vi "write_params.vi"(8 "error in (no error)":errorcluster, 10 "params":T1={"n_components"=2.0, "algorithm"="randomized", "n_iter"=5.0, "random_state"=0.0, "tol"=0.0}, 11 "TruncatedSVD in":refnum<class "TruncatedSVD.lvclass">) -> (0 "error out":errorcluster, 3 "TruncatedSVD out":refnum<class "TruncatedSVD.lvclass">)   [LabVIEW 2020, in "TruncatedSVD.lvclass"]
uses:
  TruncatedSVD.lvclass
  Controls/truncated_svd_params.ctl
  TruncatedSVD.lvclass/TruncatedSVD.ctl
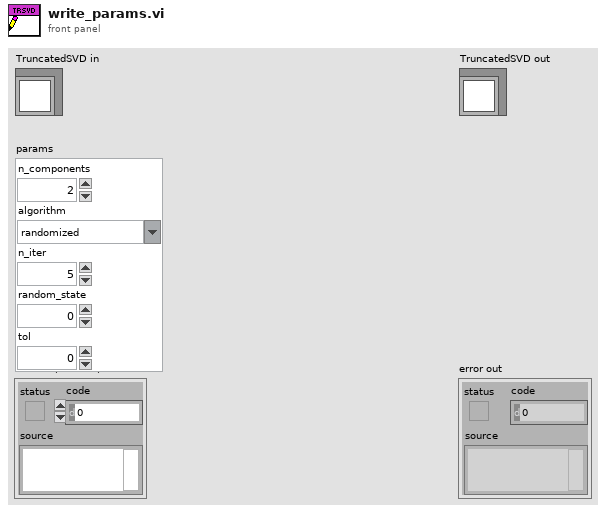
[diagram p1: front panel]
types:
  T1 = typedef "truncated_svd_params.ctl" = cluster{"n_components":dbl, "algorithm":string, "n_iter":dbl, "random_state":dbl, "tol":dbl}
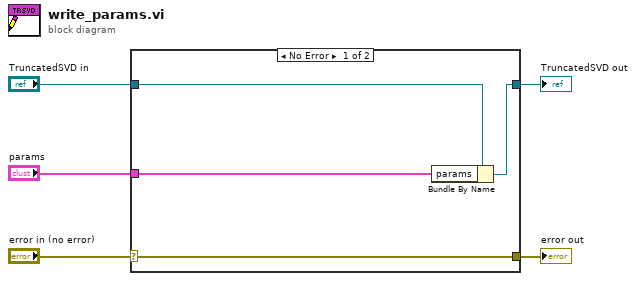
[diagram p0: block diagram]
diagram:
  n1 = case shown="No Error" "error in (no error)" {
    selector: "error in (no error)" -> [w9 w10]
    tunnel: [w9 w10] -> w4
    tunnel: [w7 w11] -> w2
    tunnel: "TruncatedSVD in" -> [w8 w11]
    tunnel: "params" -> [w6 _]
    frame No Error {
      n2 = Bundle By Name(cluster=w8, "params"=w6) -> (w7:refnum<class "TruncatedSVD.lvclass">)
    }
    frame Error {
    }
  }
  "error out" <- w4
  "TruncatedSVD out" <- w2
